vi "Read Serial Number.vi"(0 "Session Handle in":T1, 11 "error in (no error)":errorcluster) -> (4 "Session Handle out":T1, 6 "Serial Number":string, 15 "error out":errorcluster)   [LabVIEW 2015, in "PAS.lvclass"]
uses:
  PAS.lvclass
  Typedefs/Session Handle.ctl
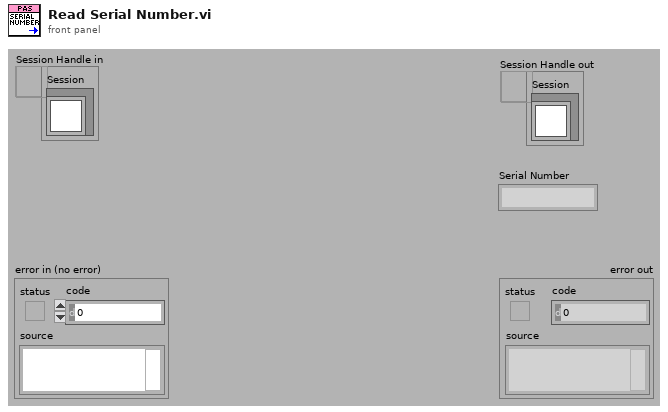
[diagram p1: front panel]
types:
  T1 = typedef "PAS.lvclass/Session Handle.ctl" = refnum<data-value>
  T2 = typedef "XNET Frame CAN.ctl" = cluster{"timestamp":timestamp, "payload":u8[], "identifier":u32, "type":T3, "extended?":bool, "echo?":bool}
  T3 = typedef "XNET Frame Type CAN.ctl" = u8
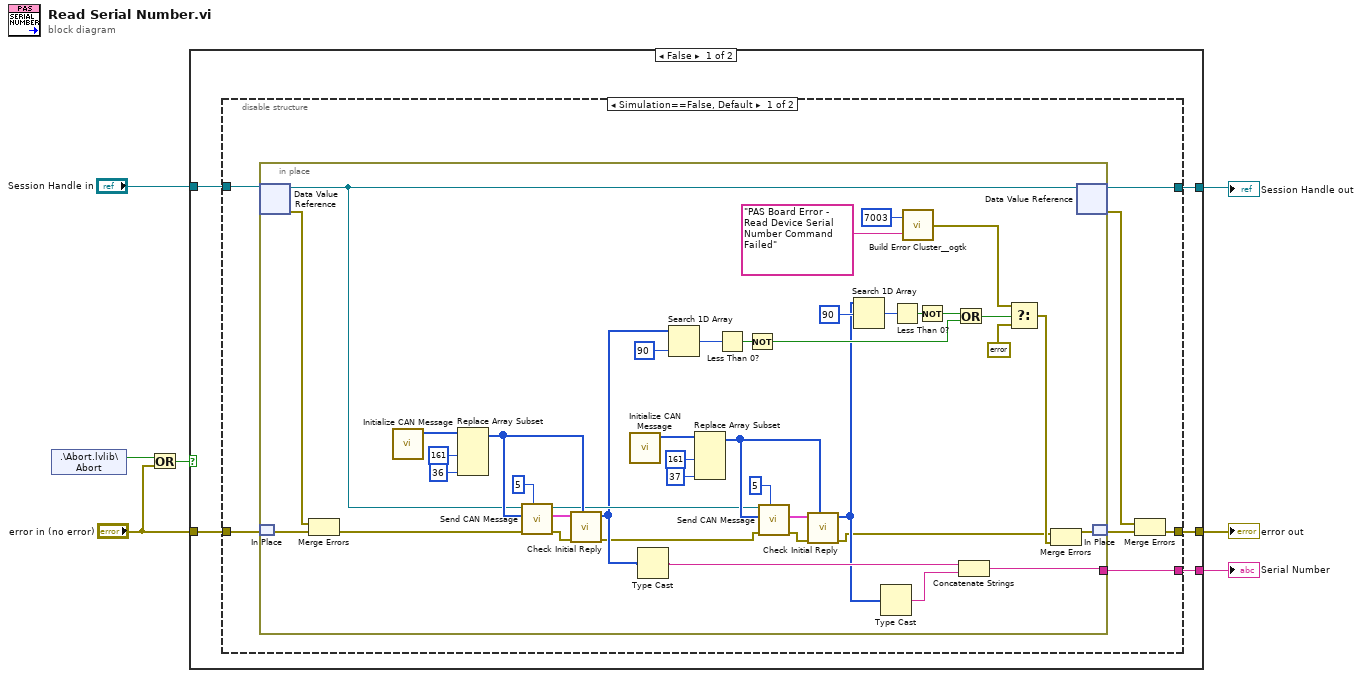
[diagram p0: block diagram]
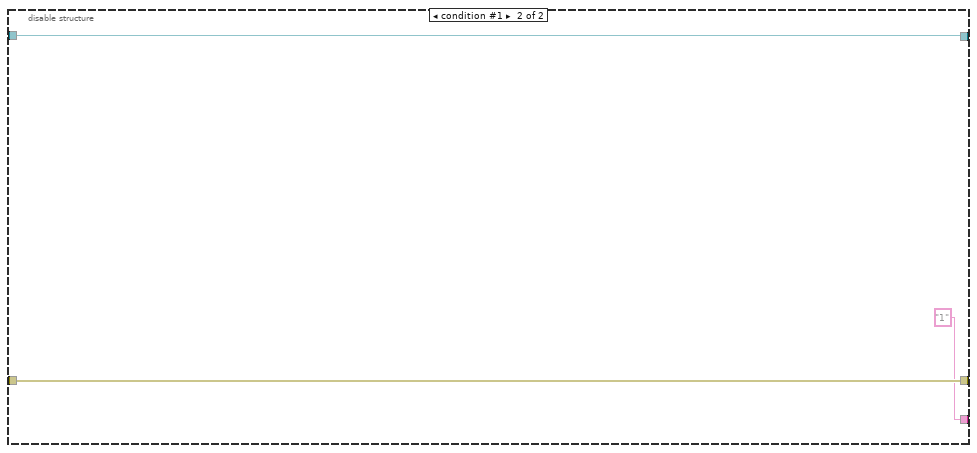
[diagram p2: hidden frame]
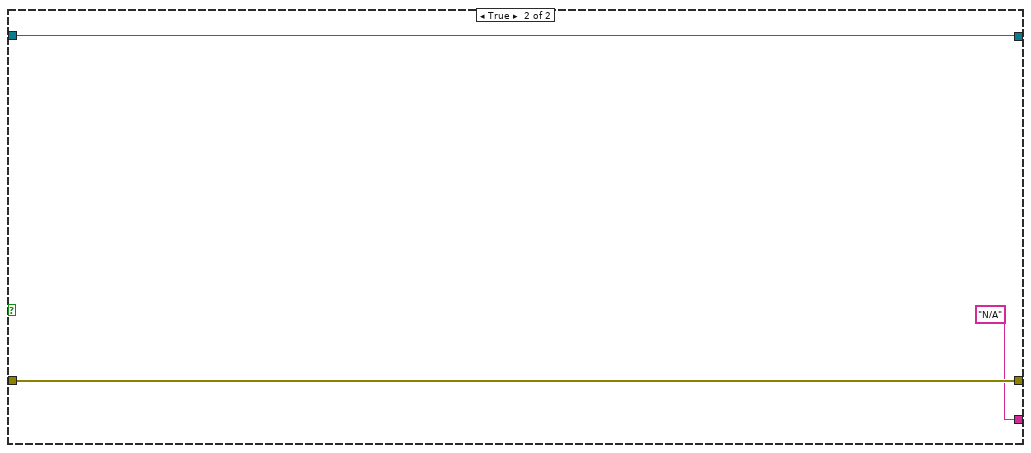
[diagram p3: hidden frame]
diagram:
  n1 = shared-variable ".\\Abort.lvlib\\Abort"() -> (w4:bool)  [unwired: 1 in, 1 out]
  n2 = Or(x=w4, y="error in (no error)") -> (x .or. y?=w2:bool)
  n3 = case shown="False" w2 {
    tunnel: [w12 w66] -> w6
    tunnel: [w11 w65] -> w5
    tunnel: "Session Handle in" -> [w10 w66]
    tunnel: "error in (no error)" -> [w9 w65]
    tunnel: [w8 "N/A"] -> w1
    frame False {
      n4 = disable-structure shown="Simulation==False, Default" {
        disable-tunnel: [w19 w63] -> w12
        disable-tunnel: [w16 w62] -> w11
        disable-tunnel: w10 -> [w15 w63]
        disable-tunnel: w9 -> [w14 w62]
        disable-tunnel: [w13 "1"] -> w8
        frame condition #0 (active) {
          n5 = in-place {
            in-place-border: [w36] -> w13
            n6 = in-place-dvr #1(w15) -> (w37:refnum<class "PAS.lvclass">, w59:errorcluster)
            n7 = in-place-match #2(w14) -> (w58:errorcluster)
            n8 = Merge Errors(w59, w58) -> (w38:errorcluster)
            n9 = call "Initialize CAN Message.vi"() -> ("Initial Payload"=w57:u8[])  [unwired: 11 in]
            n10 = Replace Array Subset(array=w57, new element #1=u8 161 ("new element/subarray"), new element #2=u8 36 ("new element/subarray")) -> (w52:u8[])  [unwired: 2 in]
            n11 = call "Send CAN Message.vi"("Number of Retries"=5, "error in (no error)"=w38, "payload"=w52, "Pas In"=w37) -> ("error out"=w23:errorcluster, "Reply"=w53:T2[], "Pas Out"=w45:refnum<class "PAS.lvclass">)  [unwired: 5 in]
            n12 = call "Check Initial Reply.vi"("Write Message"=w52, "error in (no error)"=w23, "Reply"=w53) -> ("error out"=w22:errorcluster, "Data Packet"=w28:u8[])  [unwired: 5 in, 2 out]
            n13 = call "Initialize CAN Message.vi"() -> ("Initial Payload"=w46:u8[])  [unwired: 11 in]
            n14 = Type Cast(x=w28) -> (*(type *) &x=w27:string)  [unwired: 1 in]
            n15 = Search 1D Array(1D array=w28, element=u8 90 ("new element/subarray")) -> (index of element=w43:i32)  [unwired: 1 in]
            n16 = Replace Array Subset(array=w46, new element #1=u8 161 ("new element/subarray"), new element #2=u8 37 ("new element/subarray")) -> (w51:u8[])  [unwired: 2 in]
            n17 = Less Than 0?(x=w43) -> (x < 0?=w39:bool)
            n18 = Not(x=w39) -> (.not. x?=w30:bool)
            n19 = call "Send CAN Message.vi"("Number of Retries"=5, "error in (no error)"=w22, "payload"=w51, "Pas In"=w45) -> ("error out"=w21:errorcluster, "Reply"=w50:T2[])  [unwired: 5 in, 1 out]
            n20 = call "Check Initial Reply.vi"("Write Message"=w51, "error in (no error)"=w21, "Reply"=w50) -> ("error out"=w20:errorcluster, "Data Packet"=w26:u8[])  [unwired: 5 in, 2 out]
            n21 = Search 1D Array(1D array=w26, element=u8 90 ("new element/subarray")) -> (index of element=w42:i32)  [unwired: 1 in]
            n22 = Type Cast(x=w26) -> (*(type *) &x=w25:string)  [unwired: 1 in]
            n23 = Less Than 0?(x=w42) -> (x < 0?=w40:bool)
            n24 = call <userlib>:"Build Error Cluster__ogtk.vi"("String to Prepend to source (\"\")"="PAS Board Error - Read Device Serial Number Command Failed" ("string"), "code"=7003) -> ("error out"=w32:errorcluster)
            n25 = Not(x=w40) -> (.not. x?=w29:bool)
            n26 = Or(x=w29, y=w30) -> (x .or. y?=w33:bool)
            n27 = Concatenate Strings(w27, w25) -> (w36:string)
            n28 = Select(t=w32, s=w33, f=errorcluster {"status"=FALSE, "code"=0, "source"=""}) -> (s? t:f=w24:errorcluster)
            n29 = Merge Errors(w20, w24) -> (w60:errorcluster)
            n30 = in-place-dvr #1(w37) -> (w19:T1, w17:errorcluster)
            n31 = in-place-match #2(w60) -> (w18:errorcluster)
          }
          n32 = Merge Errors(w17, w18) -> (w16:errorcluster)
        }
        frame condition #1 {
        }
      }
    }
    frame True {
    }
  }
  "Session Handle out" <- w6
  "error out" <- w5
  "Serial Number" <- w1
